vi "NEW数据采集传输系统.vi"() -> ()   [LabVIEW 2016, in "数据传输系统.lvlib"]
uses:
  <vilib>/Utility/miscctls.llb/LVPointTypeDef.ctl
  <vilib>/Utility/error.llb/whitespace.ctl
  <vilib>/picture/picture.llb/imagedata.ctl
  <vilib>/Utility/config.llb/NI_LVConfig.lvlib
  update/update.lvlib
panel:
  in  "串口透传":bool
  in  "共享MN":bool
  out "剖面数据补发":bool
  out "日志信息补发":bool
  out "数据补发":bool
  in  "自动更新":bool
  in  "数据补传":bool caption="确定"
  out "数据库打开失败次数":dbl
  out "与工控通信指示灯":bool
  in  "判断数据反馈":enum16{"非严格判断", "严格判断", "不判断"}(ring)
  in  "暂停上传":bool
  in  "配置表":bool caption="确定"
  in  "updateconfiguration":T1={"主机"="27.154.58.30", "用户"="update", "密码"="std23506", "远程路径"="数据传输系统\\平台数据传输系统.exe", "下载文件名"="平台数据传输系统.exe", "软件版本"=""}
  out "标题显示":string
  in  "更新":bool
  in  "系统编码选择框":string(combo)="地表水质量监测"
  in  "数据发送通道":enum16{"TCP", "VISA"}(ring)
  in  "baud rate":u32=9600 caption="波特率"
  in  "VISA resource name":refnum<visa-resource-name> caption="VISA资源名称"
  in  "实时数据发送时间间隔/min":i32=1
  in  "数据组合发送":bool
  in  "2011发送":bool
  in  "数据发送协议":enum16{"2005-212协议", "2017-212协议"}(ring)=enum."2017-212协议"
  in  "重发时间":T2(ring)
  in  "重发日期":T3(ring)
  in  "开机启动":bool
  in  "每周自动重发":bool=TRUE
  in  "确定":bool
  in  "返回":bool
  in  "PW":string
  in  "MN":string
  in  "PORT":string
  in  "IP":string
  in  "站点设备":string
  in  "站点名称":string
  out "设置超时时间/min":i32=1
  out "状态信息":T4={"1st Error to Convert "=63, "步骤 "=enum."发送数据", "元素"="实时数据", "TCP服务端掉线计数"=0, "TCP掉线时间节点"="2019/05/08 15:24:17"} {"1st Error to Convert" items=["无错误", "参数错误", "内存已满", "超出区域", "文件结束", "文件已打开", "一般文件IO错误", "未找到文件", "文件权限错误", "磁盘已满", "路径副本", "打开过多文件", "未启用", "未找到资源文件", "无法添加资源", "未找到资源", "未找到图像", "图像内存错误", "画笔不存在", "配置错误类型", "配置未找到解析段", "配置解析错误", "配置内存错误", "错误外部代码格式", "错误外部代码偏移量", "外部代码不存在", "空窗口", "销毁窗口错误", "空菜单", "打印已中止", "错误打印记录", "打印驱动程序错误", "打印时窗口错误", "打印时内存错误", "打印对话框错误", "一般打印错误", "无效设备引用句柄", "设备未找到", "设备参数错误", "设备单位错误", "无法打开设备", "设备调用已中止", "一般错误", "用户已取消", "对象ID过低", "对象ID过高", "对象不在堆中", "未知的堆", "错误DefProc ID", "DefProc不在表格中", "范围外信息", "空方法", "未知信息", "不支持管理器调用", "错误地址", "连接过程中", "连接超时", "连接过程中", "不支持网络属性", "网络错误", "正在使用的地址", "系统缺少内存", "连接已中止", "连接已拒绝", "连接未建立", "连接已建立", "连接已关闭", "初始化错误（交互应用程序管理器）", "错误事件发生", "等待无约束事件发生处理程序", "事件发生队列溢出", "错误路径", "未发出信号量", "未识别类型（交互应用程序管理器）"]}
  out "数据接收超时指示灯":bool
  out "空闲时间/s":string
  out "系统时间":string
  out "实时小时数据上传":bool
  out "系统状态改变":bool
  out "软件版本":string
  out "掉线指示":bool
  out "核查数据上传":bool
  out "配置信息":T5
  in  "参数配置":bool
  out "反控数据发送":bool
  out "读取报文显示":string
  out "发送报文显示":string
  out "心跳包":bool
  out "通信状态":bool
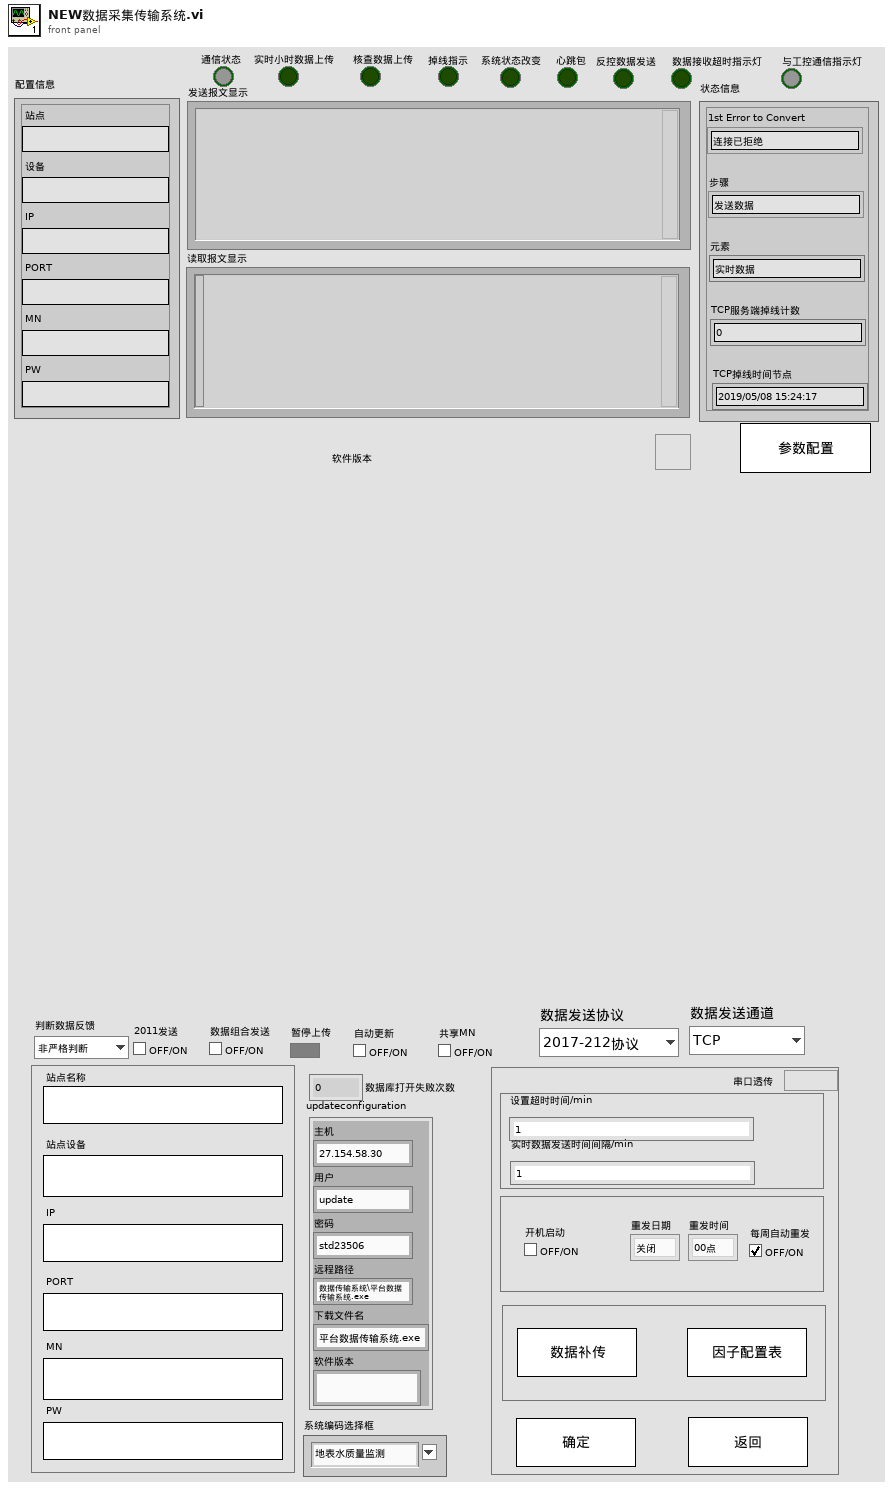
[diagram p1: front panel]
types:
  T1 = cluster{"主机":string, "用户":string, "密码":string, "远程路径":string, "下载文件名":string, "软件版本":string}
  T2 = enum16{"00点", "01点", "02点", "03点", "04点", "05点", "06点", "07点", "08点", "09点", "10点", "11点", "12点", "13点", "14点", "15点", "16点", "17点", "18点", "19点", "20点", "21点", "22点", "23点"}
  T3 = enum16{"关闭", "星期日", "星期一", "星期二", "星期三", "星期四", "星期五", "星期六"}
  T4 = cluster{"1st Error to Convert ":i32, "步骤 ":enum16{"打开连接", "发送数据", "读取数据", "数据处理", "关闭连接"}, "元素":string, "TCP服务端掉线计数":i32, "TCP掉线时间节点":string}
  T5 = cluster{"站点":string, "设备":string, "IP":string, "PORT":string, "MN":string, "PW":string}
  T6 = typedef "imagedata.ctl" = cluster{"image type":i32, "image depth":i32, "image":u8[], "mask":u8[], "colors":u32[], "Rectangle":cluster{"left":i16, "top":i16, "right":i16, "bottom":i16}}
  T7 = typedef "LVPointTypeDef.ctl" = cluster{"Horizontal":i16, "Vertical":i16}
  T8 = cluster{"setini":string, "sysini":string, "hechaini":string, "actualwrite":string, "actualread":string, "datasent":string, "反控命令信息队列":string, "反控与仪器交互":string}
  T9 = cluster{"配置表格[0]":string, "配置表格[1]":string, "配置表格[2]":string, "配置表格[3]":string, "配置表格[4]":string, "配置表格[5]":string, "配置表格[6]":string, "配置表格[7]":string, "配置表格[8]":string, "配置表格[9]":string, "配置表格[10]":string, "配置表格[11]":string, "配置表格[12]":string, "配置表格[13]":string, "配置表格[14]":string, "配置表格[15]":string, "配置表格[16]":string, "配置表格[17]":string, "配置表格[18]":string, "配置表格[19]":string, "配置表格[20]":string, "配置表格[21]":string, "配置表格[22]":string, "配置表格[23]":string, "配置表格[24]":string, "配置表格[25]":string, "配置表格[26]":string, "配置表格[27]":string, "配置表格[28]":string, "配置表格[29]":string, "配置表格[30]":string, "配置表格[31]":string, "配置表格[32]":string, "配置表格[33]":string, "配置表格[34]":string, "配置表格[35]":string, "配置表格[36]":string, "配置表格[37]":string}
  T10 = cluster{"[0]":dbl, "[1]":dbl, "[2]":dbl, "[3]":dbl, "[4]":dbl, "[5]":dbl, "[6]":dbl, "[7]":dbl, "[8]":dbl, "[9]":dbl, "[10]":dbl, "[11]":dbl, "[12]":dbl, "[13]":dbl, "[14]":dbl, "[15]":dbl, "[16]":dbl, "[17]":dbl, "[18]":dbl, "[19]":dbl, "[20]":dbl, "[21]":dbl, "[22]":dbl, "[23]":dbl, "[24]":dbl, "[25]":dbl, "[26]":dbl, "[27]":dbl, "[28]":dbl, "[29]":dbl, "[30]":dbl, "[31]":dbl, "[32]":dbl, "[33]":dbl, "[34]":dbl, "[35]":dbl, "[36]":dbl, "[37]":dbl}
  T11 = cluster{"时间标识":timestamp, "设备":string, "日志信息":string, "流程参数":string}
  T12 = typedef "NI_LVConfig.lvlib/Config Data RefNum.ctl" = refnum<k1>
  T13 = cluster{"CODMn":bool, "CODCr":bool, "DO":bool, "铜":bool, "PH":bool, "氨氮":bool, "比电导率":bool, "水温":bool, "COD":bool, "浊度":bool, "总氮":bool, "总磷":bool, "叶绿素a":bool, "藻密度":bool, "水位":bool, "流速":bool, "瞬时流量":bool, "累积流量":bool, "亚硝氮":bool, "硫化物":bool, "ORP":bool, "铅":bool, "镉":bool, "锌":bool, "镍":bool, "锰":bool, "汞":bool, "气温":bool, "气压":bool, "风速":bool, "风向":bool, "盐度":bool, "磷酸盐":bool, "硝氮":bool, "氟化物":bool, "挥发酚":bool, "氯化物":bool}
  T14 = cluster{"time1":string, "time2":string, "time3":string, "time4":string, "time5":string, "time6":string, "time7":string, "time8":string, "time9":string, "time10":string, "time11":string, "time12":string, "time13":string, "time14":string, "time15":string, "time16":string, "time17":string, "time18":string, "time19":string, "time20":string, "time21":string, "time22":string, "time23":string, "time24":string, "time25":string, "time26":string, "time27":string, "time28":string, "time29":string, "time30":string, "time31":string, "time32":string, "time33":string, "time34":string, "time35":string, "time36":string, "time37":string}
  T15 = cluster{"[0]":string, "[1]":string, "[2]":string, "[3]":string, "[4]":string, "[5]":string, "[6]":string, "[7]":string}
  T16 = cluster{"[0]":string, "[1]":string, "[2]":string, "[3]":string, "[4]":string, "[5]":string, "[6]":string, "[7]":string, "[8]":string, "[9]":string}
  T17 = cluster{"[0]":string, "[1]":string, "[2]":string, "[3]":string, "[4]":string, "[5]":string, "[6]":string}
  T18 = cluster{"[0]":string, "[1]":string, "[2]":string, "[3]":string, "[4]":string, "[5]":string, "[6]":string, "[7]":string, "[8]":string, "[9]":string, "[10]":string, "[11]":string, "[12]":string, "[13]":string, "[14]":string, "[15]":string, "[16]":string, "[17]":string}
  T19 = cluster{"[0]":string, "[1]":string, "[2]":string, "[3]":string, "[4]":string, "[5]":string, "[6]":string, "[7]":string, "[8]":string, "[9]":string, "[10]":string, "[11]":string, "[12]":string, "[13]":string, "[14]":string}
  T20 = cluster{"[0]":string, "[1]":string, "[2]":string, "[3]":string, "[4]":string, "[5]":string, "[6]":string, "[7]":string, "[8]":string, "[9]":string, "[10]":string, "[11]":string, "[12]":string, "[13]":string, "[14]":string, "[15]":string, "[16]":string, "[17]":string, "[18]":string, "[19]":string, "[20]":string, "[21]":string, "[22]":string, "[23]":string, "[24]":string, "[25]":string, "[26]":string, "[27]":string, "[28]":string, "[29]":string, "[30]":string, "[31]":string, "[32]":string, "[33]":string, "[34]":string, "[35]":string, "[36]":string}
  T21 = typedef "whitespace.ctl" = u16
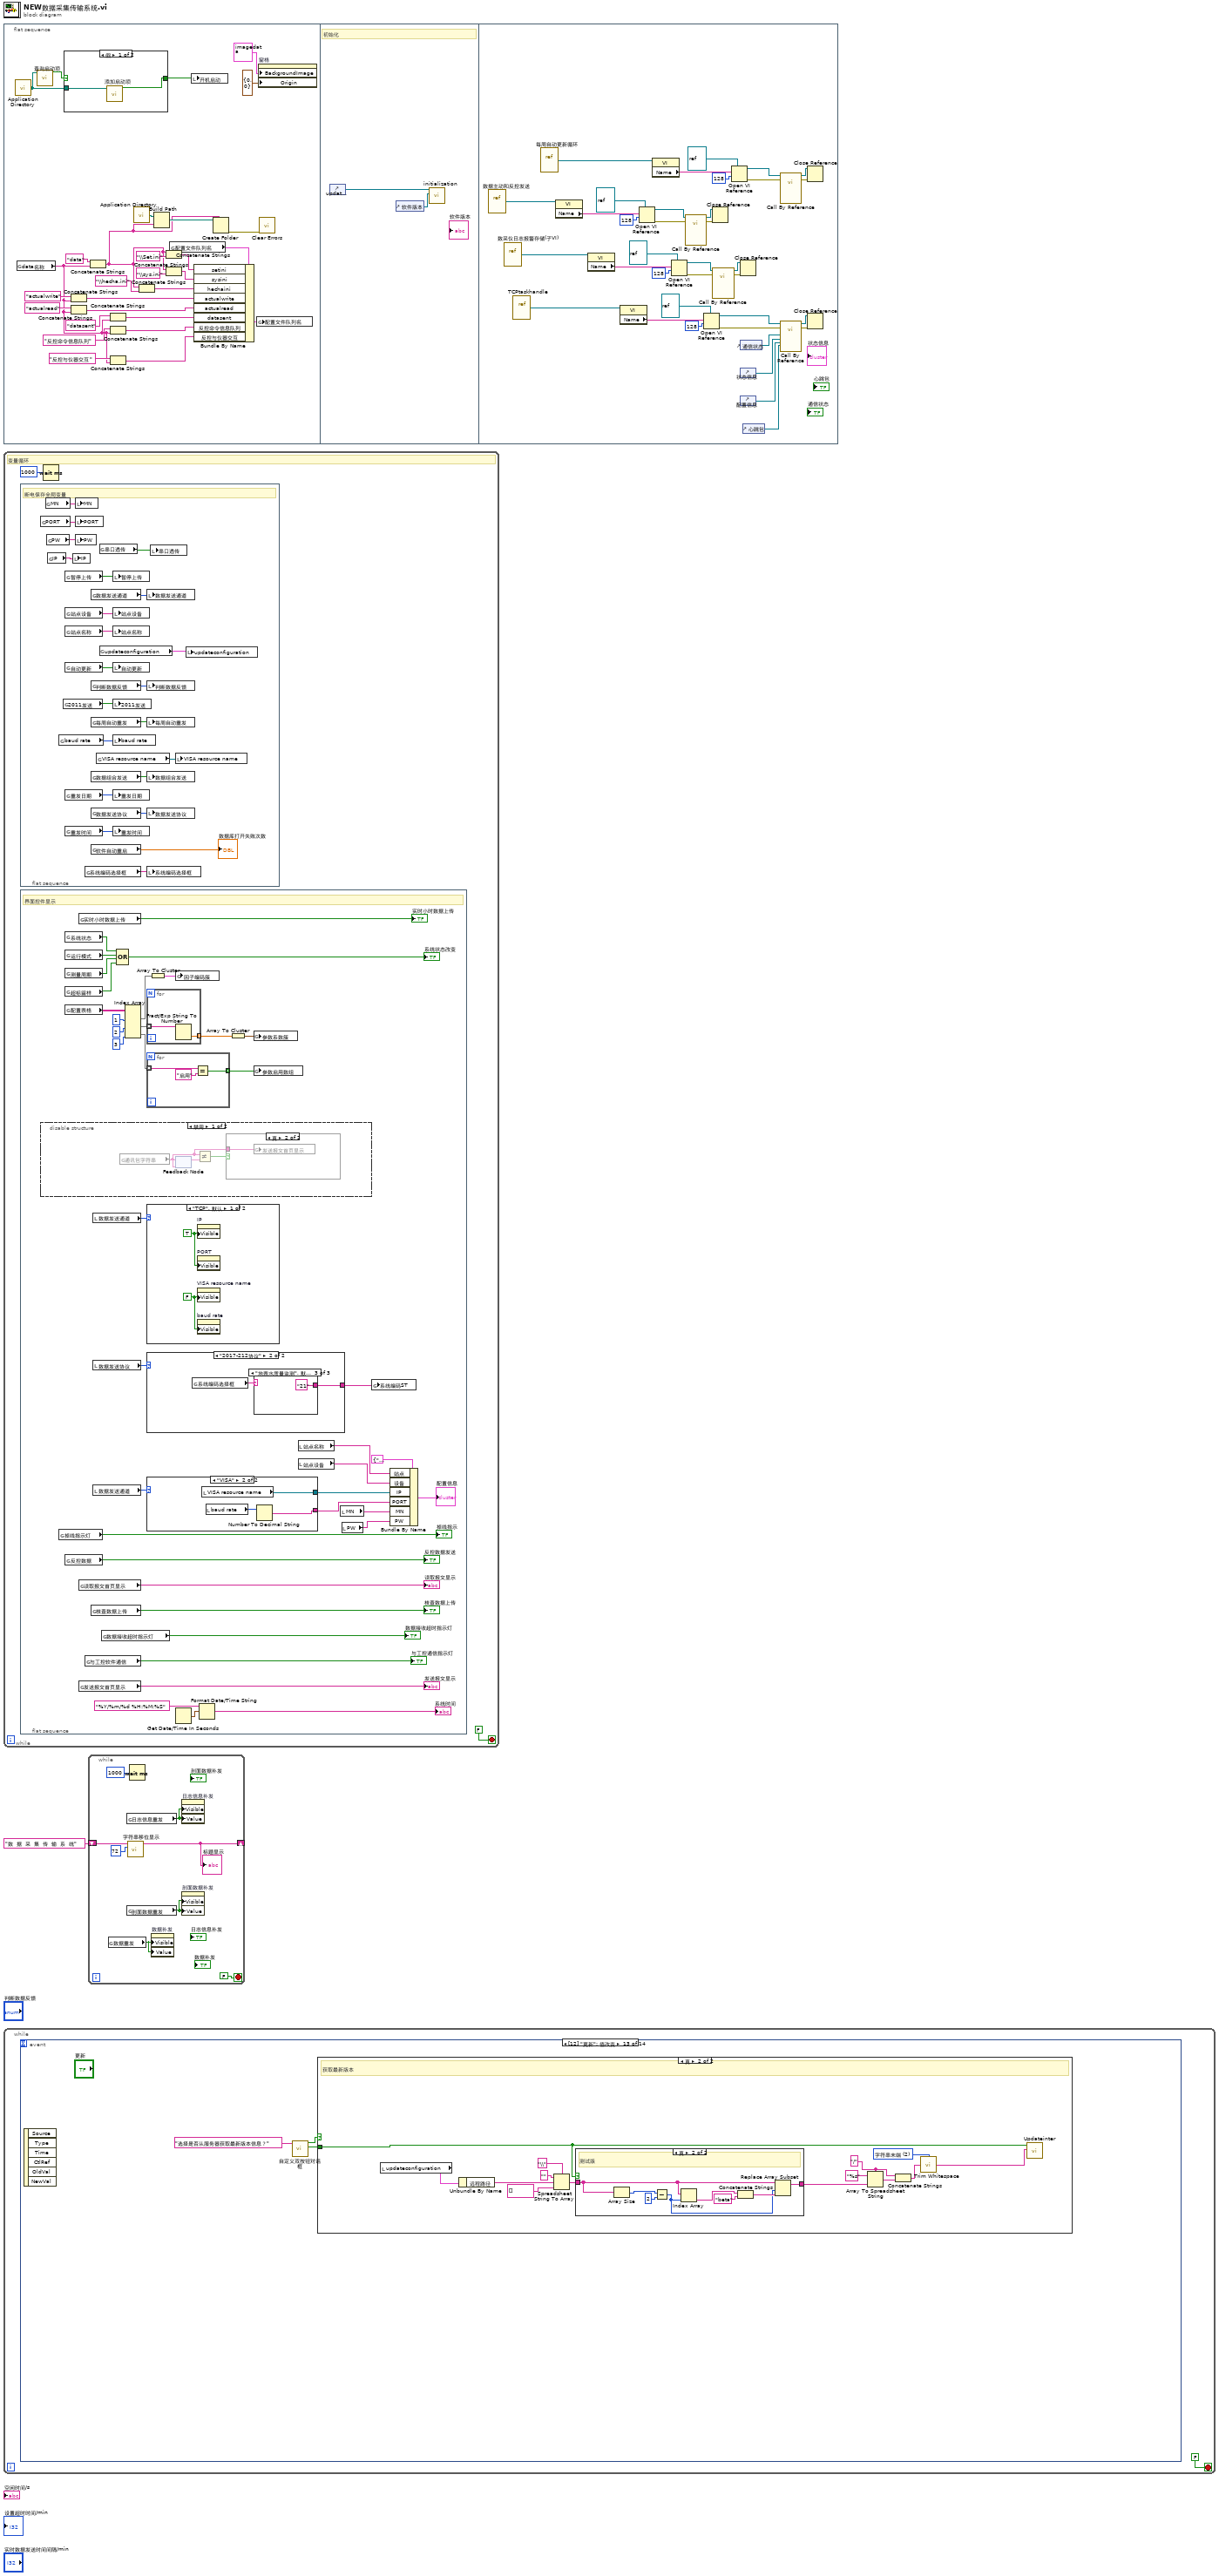
[diagram p0: block diagram]
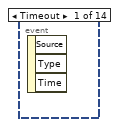
[diagram p2: hidden frame]
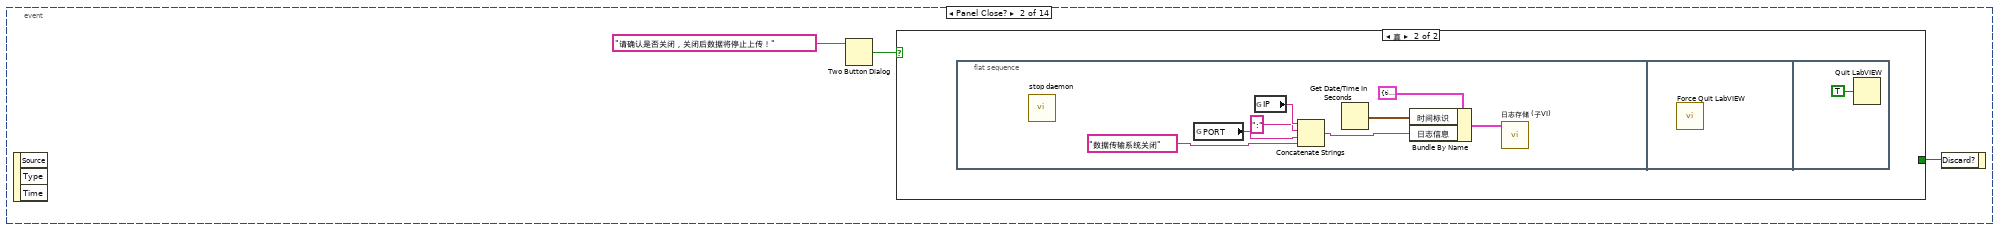
[diagram p3: hidden frame]
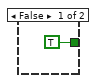
[diagram p4: hidden frame]
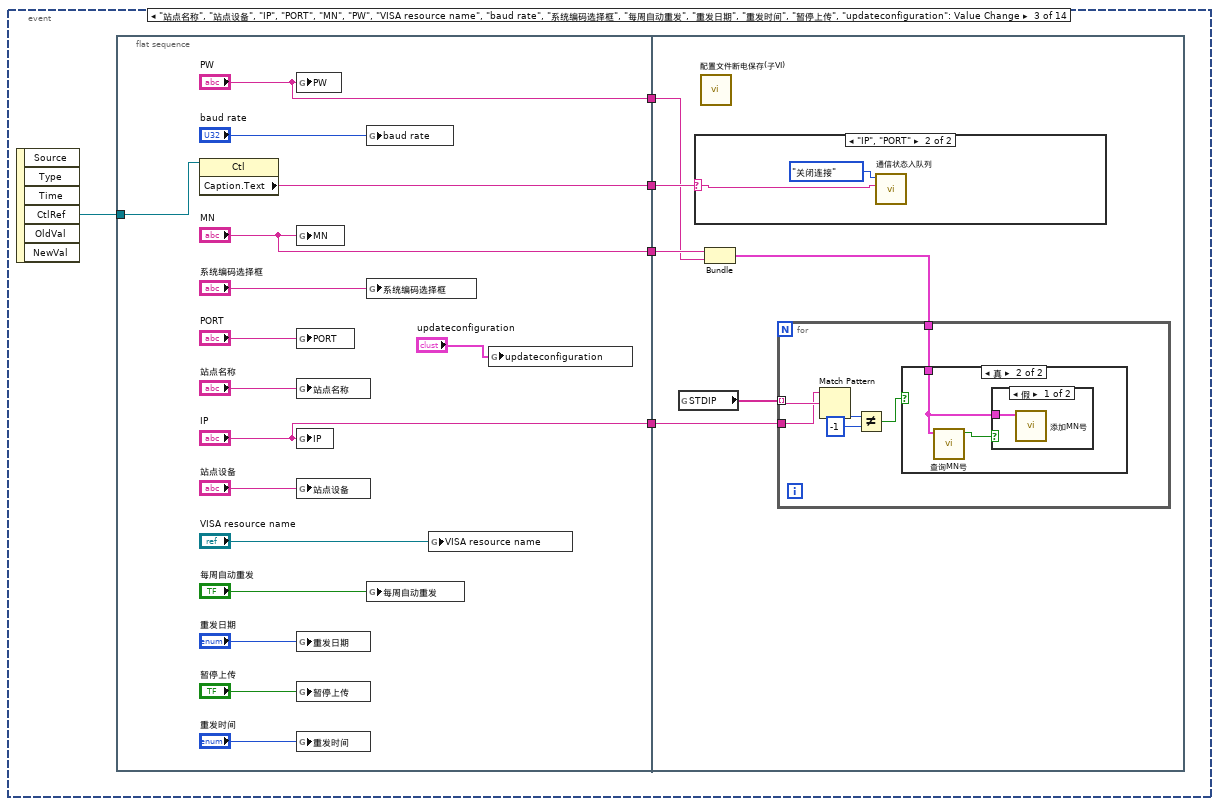
[diagram p5: hidden frame]
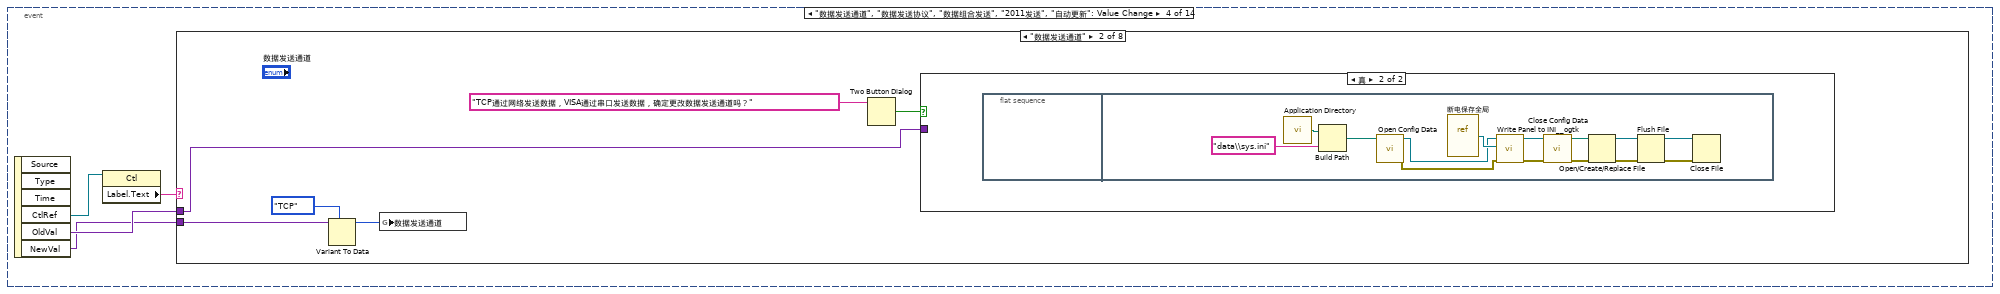
[diagram p9: hidden frame]
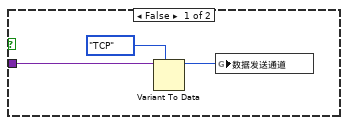
[diagram p11: hidden frame]
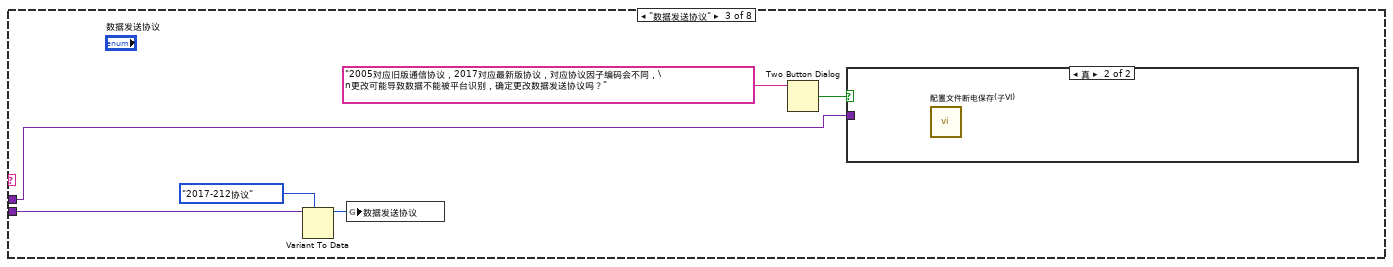
[diagram p12: hidden frame]
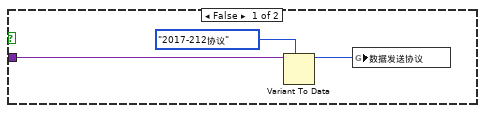
[diagram p13: hidden frame]
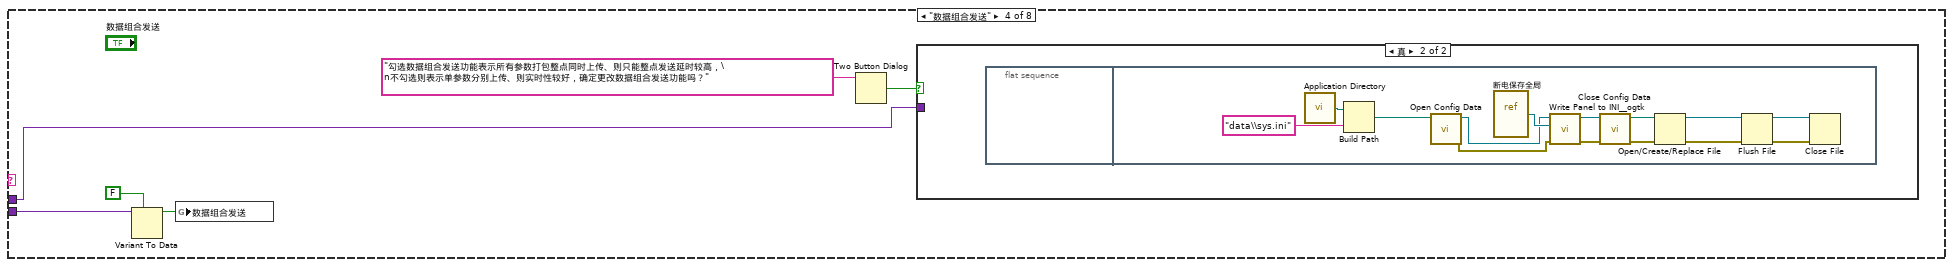
[diagram p14: hidden frame]
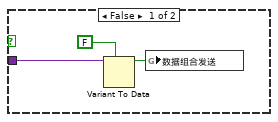
[diagram p15: hidden frame]
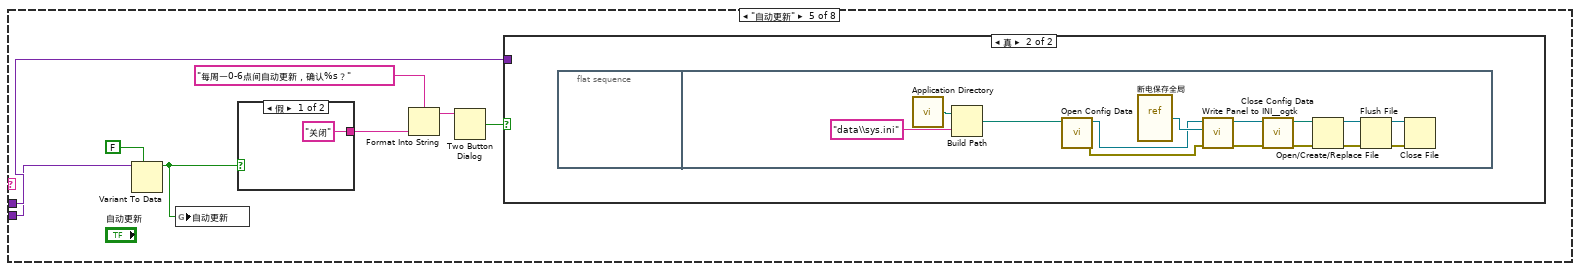
[diagram p16: hidden frame]
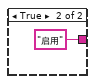
[diagram p17: hidden frame]
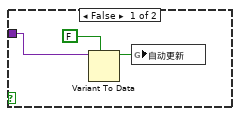
[diagram p18: hidden frame]
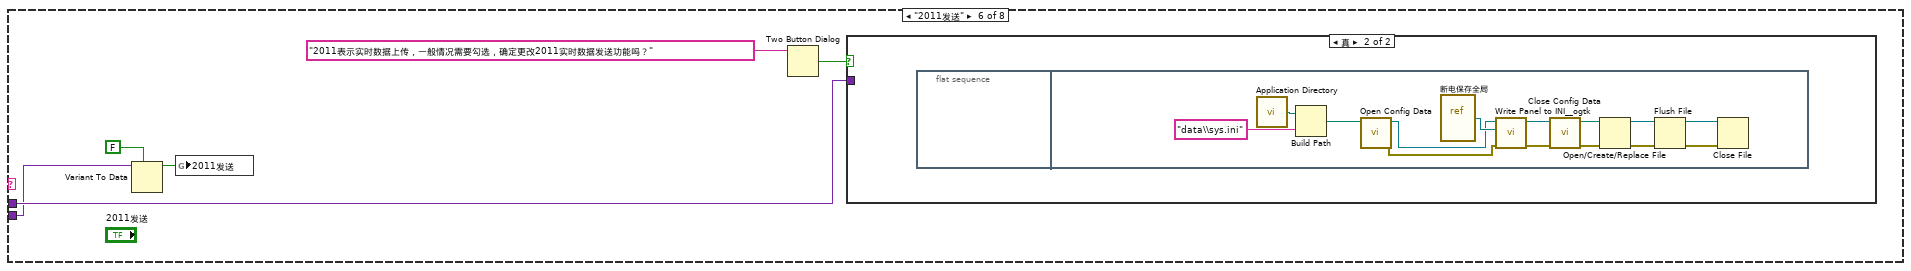
[diagram p19: hidden frame]
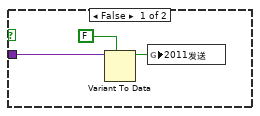
[diagram p20: hidden frame]
diagram:
  n1 = flat-sequence {
    frame #0 {
      n2 = call <vilib>:"Application Directory.vi"() -> ("Application Directory"=w8:path)
      n3 = global read "断电保存全局.vi" "data名称"() -> (w4:string)
      n4 = call "查询启动项.vi"("启动文件路径"=w8) -> ("包含启动项"=w7:bool)  [unwired: 9 in, 1 out]
      n5 = case shown="假" w7 {
        selector: w7 -> [_ w33]
        tunnel: w8 -> [w32 _]
        tunnel: [w31 w33] -> w6
        frame False {
          n6 = call "添加启动项.vi"("启动文件路径"=w32) -> ("添加成功标记"=w31:bool)  [unwired: 9 in, 1 out]
        }
        frame True {
        }
      }
      n7 = Concatenate Strings("actualwrite" ("名称（未命名）"), w4) -> (w18:string)
      n8 = Concatenate Strings("actualread" ("名称（未命名）"), w4) -> (w16:string)
      n9 = Concatenate Strings("data" ("对话框窗口（创建文件夹）"), w4) -> (w23:string)
      n10 = Concatenate Strings("datasent" ("名称（未命名）"), w4) -> (w14:string)
      n11 = Concatenate Strings("反控命令信息队列" ("名称（未命名）"), w4) -> (w10:string)
      n12 = Concatenate Strings("反控与仪器交互" ("名称（未命名）"), w4) -> (w11:string)
      n13 = call <vilib>:"Application Directory.vi"() -> ("Application Directory"=w29:path)
      n14 = Concatenate Strings(w23, "\\hecha.ini" ("名称或相对路径")) -> (w21:string)
      n15 = Build Path(base path=w29, name or relative path=w23) -> (appended path=w28:path)
      n16 = Concatenate Strings(w23, "\\Set.ini" ("名称或相对路径")) -> (w25:string)
      n17 = Concatenate Strings(w23, "\\sys.ini" ("名称或相对路径")) -> (w22:string)
      n18 = global read "全局1.vi" "配置文件队列名"() -> (w2:T8)
      n19 = local write "开机启动"(w6) -> ()
      n20 = Bundle By Name(cluster=w2, "setini"=w25, "sysini"=w22, "hechaini"=w21, "actualwrite"=w18, "actualread"=w16, "datasent"=w14, "反控命令信息队列"=w10, "反控与仪器交互"=w11) -> (w3:T8)
      n21 = Create Folder(prompt (Create Folder)=w23, path (use dialog)=w28) -> (error out=w27:errorcluster)  [unwired: 1 in, 2 out]
      n22 = global write "全局1.vi" "配置文件队列名"(w3) -> ()
      n23 = property on="窗格" class="Pane"("BackgroundImage"=T6 {"image type"=0, "image depth"=24, "image"=array[12288000 elements], "mask"=[], "colors"=[], "Rectangle"={"left"=0, "top"=0, "right"=2560, "bottom"=1600}} ("image data"), "Origin"=T7 {"Horizontal"=0, "Vertical"=0} ("原点")) -> ()  [unwired: 2 in, 2 out]
      n24 = call <vilib>:"Clear Errors.vi"("error in (no error)"=w27) -> ()  [unwired: 5 in, 2 out]
    }
    frame #1 {
      # "初始化"
      n25 = control-ref of="updateconfiguration"() -> (w35:refnum<vi>)
      n26 = control-ref of="软件版本"() -> (w34:refnum<vi>)
      n27 = call "initialization.vi"("软件版本"=w34, "updateconfiguration"=w35) -> ()  [unwired: 9 in]
    }
    frame #2 {
      n28 = vi-ref "数据主动和反控发送.vi"() -> (w63:refnum<vi>)
      n29 = vi-ref "数采仪日志报警存储(子VI).vi"() -> (w64:refnum<vi>)
      n30 = vi-ref "TCPtaskhandle.vi"() -> (w40:refnum<vi>)
      n31 = vi-ref "每周自动更新循环.vi"() -> (w55:refnum<vi>)
      n32 = property class="VI"(reference=w63) -> ("Name"=w62:string)  [unwired: 1 in, 2 out]
      n33 = property class="VI"(reference=w64) -> ("Name"=w71:string)  [unwired: 1 in, 2 out]
      n34 = property class="VI"(reference=w40) -> ("Name"=w47:string)  [unwired: 1 in, 2 out]
      n35 = Open VI Reference(type specifier VI Refnum (for type only)=refnum<vi> refnum, vi path=w62, options=128 ("选项")) -> (vi reference=w60:refnum<vi>, error out=w58:errorcluster)  [unwired: 3 in]
      n36 = property class="VI"(reference=w55) -> ("Name"=w48:string)  [unwired: 1 in, 2 out]
      n37 = Open VI Reference(type specifier VI Refnum (for type only)=refnum<vi> refnum, vi path=w71, options=128 ("选项")) -> (vi reference=w69:refnum<vi>, error out=w67:errorcluster)  [unwired: 3 in]
      n38 = call-by-ref "?"(reference=w60, error in=w58) -> (reference out=w56:refnum<vi>, error out=w57:errorcluster)  [unwired: 12 in]
      n39 = Open VI Reference(type specifier VI Refnum (for type only)=refnum<vi> refnum, vi path=w47, options=128 ("选项")) -> (vi reference=w45:refnum<vi>, error out=w43:errorcluster)  [unwired: 3 in]
      n40 = Close Reference(reference=w56, error in (no error)=w57) -> ()  [unwired: 1 out]
      n41 = call-by-ref "?"(reference=w69, error in=w67) -> (reference out=w65:refnum<vi>, error out=w66:errorcluster)  [unwired: 12 in]
      n42 = Open VI Reference(type specifier VI Refnum (for type only)=refnum<vi> refnum, vi path=w48, options=128 ("选项")) -> (vi reference=w50:refnum<vi>, error out=w52:errorcluster)  [unwired: 3 in]
      n43 = Close Reference(reference=w65, error in (no error)=w66) -> ()  [unwired: 1 out]
      n44 = control-ref of="通信状态"() -> (w39:refnum<vi>)
      n45 = control-ref of="状态信息"() -> (w38:refnum<vi>)
      n46 = control-ref of="配置信息"() -> (w37:refnum<vi>)
      n47 = control-ref of="心跳包"() -> (w36:refnum<vi>)
      n48 = call-by-ref "?"(reference=w50, error in=w52) -> (reference out=w54:refnum<vi>, error out=w53:errorcluster)  [unwired: 12 in]
      n49 = call-by-ref "?"(reference=w45, error in=w43, "心跳包"=w36, "配置信息"=w37, "状态信息"=w38, "通信状态"=w39) -> (reference out=w41:refnum<vi>, error out=w42:errorcluster)  [unwired: 8 in]
      n50 = Close Reference(reference=w54, error in (no error)=w53) -> ()  [unwired: 1 out]
      n51 = Close Reference(reference=w41, error in (no error)=w42) -> ()  [unwired: 1 out]
    }
  }
  n52 = while {
    stop <- FALSE stop-if-true
    # "变量循环"
    n53 = flat-sequence {
      frame #0 {
        # "断电保存全局变量"
        n54 = global read "断电保存全局.vi" "PORT"() -> (w159:string)
        n55 = global read "断电保存全局.vi" "MN"() -> (w158:string)
        n56 = global read "断电保存全局.vi" "PW"() -> (w157:string)
        n57 = global read "断电保存全局.vi" "IP"() -> (w160:string)
        n58 = global read "断电保存全局.vi" "baud rate"() -> (w155:u32)
        n59 = global read "断电保存全局.vi" "2011发送"() -> (w151:bool)
        n60 = global read "断电保存全局.vi" "暂停上传"() -> (w145:bool)
        n61 = global read "断电保存全局.vi" "站点设备"() -> (w161:string)
        n62 = global read "断电保存全局.vi" "站点名称"() -> (w162:string)
        n63 = global read "断电保存全局.vi" "自动更新"() -> (w143:bool)
        n64 = global read "断电保存全局.vi" "重发日期"() -> (w153:T3)
        n65 = global read "断电保存全局.vi" "重发时间"() -> (w146:T2)
        n66 = local write "IP"(w160) -> ()
        n67 = local write "MN"(w158) -> ()
        n68 = local write "PORT"(w159) -> ()
        n69 = local write "PW"(w157) -> ()
        n70 = global read "断电保存全局.vi" "系统编码选择框"() -> (w147:string)
        n71 = global read "断电保存全局.vi" "数据发送通道"() -> (w148:enum16{"TCP", "VISA"})
        n72 = global read "断电保存全局.vi" "判断数据反馈"() -> (w152:enum16{"非严格判断", "严格判断", "不判断"})
        n73 = global read "断电保存全局.vi" "每周自动重发"() -> (w154:bool)
        n74 = global read "断电保存全局.vi" "数据组合发送"() -> (w150:bool)
        n75 = global read "断电保存全局.vi" "数据发送协议"() -> (w149:enum16{"2005-212协议", "2017-212协议"})
        n76 = global read "全局1.vi" "软件自动重启"() -> (→"数据库打开失败次数":dbl)
        n77 = global read "断电保存全局.vi" "VISA resource name"() -> (w156:refnum<visa-resource-name>)
        n78 = global read "断电保存全局.vi" "串口透传"() -> (w141:bool)
        n79 = global read "断电保存全局.vi" "updateconfiguration"() -> (w142:T1)
        n80 = local write "暂停上传"(w145) -> ()
        n81 = local write "站点设备"(w161) -> ()
        n82 = local write "站点名称"(w162) -> ()
        n83 = local write "自动更新"(w143) -> ()
        n84 = local write "2011发送"(w151) -> ()
        n85 = local write "baud rate"(w155) -> ()
        n86 = local write "重发日期"(w153) -> ()
        n87 = local write "重发时间"(w146) -> ()
        n88 = local write "数据发送通道"(w148) -> ()
        n89 = local write "判断数据反馈"(w152) -> ()
        n90 = local write "每周自动重发"(w154) -> ()
        n91 = local write "数据组合发送"(w150) -> ()
        n92 = local write "数据发送协议"(w149) -> ()
        n93 = local write "系统编码选择框"(w147) -> ()
        n94 = local write "串口透传"(w141) -> ()
        n95 = local write "VISA resource name"(w156) -> ()
        n96 = local write "updateconfiguration"(w142) -> ()
      }
    }
    n97 = flat-sequence {
      frame #0 {
        # "界面控件显示"
        n98 = disable-structure shown="禁用" {
          frame Disabled {
            n99 = global read "全局1.vi" "通讯包字符串"() -> (w114:string)
            n100 = feedback #1(w114) -> (w115:string)
            n101 = feedback-in #1(w114) -> ()
            n102 = Not Equal?(x=w114, y=w115) -> (x != y?=w113:bool)
            n103 = case shown="真" w113 {
              tunnel: w114 -> [_ w116]
              frame False {
              }
              frame True {
                n104 = global write "全局1.vi" "发送报文首页显示"(w116) -> ()
              }
            }
          }
          frame Enabled {
          }
        }
        n105 = global read "全局 数据发送重叠.vi" "掉线指示灯"() -> (→"掉线指示":bool)
        n106 = global read "全局1.vi" "系统状态"() -> (w86:bool)
        n107 = global read "全局1.vi" "运行模式"() -> (w87:bool)
        n108 = global read "全局1.vi" "测量周期"() -> (w88:bool)
        n109 = global read "全局1.vi" "超标留样"() -> (w89:bool)
        n110 = global read "断电保存全局.vi" "配置表格"() -> (w84:string[][])
        n111 = global read "全局1.vi" "反控数据"() -> (→"反控数据发送":bool)
        n112 = global read "全局1.vi" "实时小时数据上传"() -> (→"实时小时数据上传":bool)
        n113 = global read "全局1.vi" "读取报文首页显示"() -> (→"读取报文显示":string)
        n114 = global read "全局1.vi" "发送报文首页显示"() -> (→"发送报文显示":string)
        n115 = global read "全局1.vi" "与工控软件通信"() -> (→"与工控通信指示灯":bool)
        n116 = global read "全局1.vi" "核查数据上传"() -> (→"核查数据上传":bool)
        n117 = local read "数据发送通道"() -> (w94:enum16{"TCP", "VISA"})
        n118 = local read "数据发送协议"() -> (w101:enum16{"2005-212协议", "2017-212协议"})
        n119 = local read "数据发送通道"() -> (w112:enum16{"TCP", "VISA"})
        n120 = global read "全局 数据发送重叠.vi" "数据接收超时指示灯"() -> (→"数据接收超时指示灯":bool)
        n121 = Compound Arithmetic op=OR ("复合运算")(w86, w87, w88, w89) -> (→"系统状态改变":bool)
        n122 = Index Array(array=w84, index (col) #1=1 ("禁用的索引 (列)"), index (col) #2=2 ("索引 (列)"), index (col) #3=3 ("索引 (列)")) -> (element #1=w82:string[], element #2=w76:string[], element #3=w78:string[])  [unwired: 3 in]
        n123 = for {
          tunnel: w76 -> [w118] mode=indexing
          tunnel: [w117] -> w75 mode=indexing
          n124 = Fract/Exp String To Number(string=w118) -> (number=w117:dbl)  [unwired: 3 in, 1 out]
        }
        n125 = for {
          tunnel: w78 -> [w121] mode=indexing
          tunnel: [w119] -> w77 mode=indexing
          n126 = Equal?(x=w121, y="启用") -> (x = y?=w119:bool)
        }
        n127 = case shown="\"TCP\", 默认" w94 {
          frame "TCP", Default {
            w122 = TRUE ("可见")
            w123 = FALSE ("可见")
            n128 = property on="IP" class="Str"("Visible"=w122) -> ()  [unwired: 2 in, 2 out]
            n129 = property on="PORT" class="Str"("Visible"=w122) -> ()  [unwired: 2 in, 2 out]
            n130 = property on="VISA resource name" class="VISAName"("Visible"=w123) -> ()  [unwired: 2 in, 2 out]
            n131 = property on="baud rate" class="DigNum (严格)"("Visible"=w123) -> ()  [unwired: 2 in, 2 out]
          }
          frame "VISA" {
            w124 = FALSE ("可见")
            w125 = TRUE ("可见")
            n132 = property on="IP" class="Str"("Visible"=w124) -> ()  [unwired: 2 in, 2 out]
            n133 = property on="PORT" class="Str"("Visible"=w124) -> ()  [unwired: 2 in, 2 out]
            n134 = property on="VISA resource name" class="VISAName"("Visible"=w125) -> ()  [unwired: 2 in, 2 out]
            n135 = property on="baud rate" class="DigNum (严格)"("Visible"=w125) -> ()  [unwired: 2 in, 2 out]
          }
        }
        n136 = case shown="\"2017-212协议\"" w101 {
          tunnel: [w126 w131] -> w100
          frame "2005-212协议", Default {
            n137 = global read "断电保存全局.vi" "系统编码选择框"() -> (w127:string)
            n138 = case shown="\"地表水体污染源\"" w127 {
              tunnel: ["52" ("设备编码MN") "32" ("设备编码MN") "21" ("设备编码MN")] -> w126
              frame "污水排放过程监测" {
              }
              frame "地表水体污染源" {
              }
              frame "地表水质量监测", Default {
              }
            }
          }
          frame "2017-212协议" {
            n139 = global read "断电保存全局.vi" "系统编码选择框"() -> (w132:string)
            n140 = case shown="\"地表水质量监测\", 默认" w132 {
              tunnel: ["52" ("设备编码MN") "32" ("设备编码MN") "21" ("设备编码MN")] -> w131
              frame "污水排放过程监测" {
              }
              frame "地表水体污染源" {
              }
              frame "地表水质量监测", Default {
              }
            }
          }
        }
        n141 = case shown="\"VISA\"" w112 {
          tunnel: [w137 w140] -> w109
          tunnel: [w136 w138] -> w106
          frame "TCP", Default {
            n142 = local read "PORT"() -> (w136:string)
            n143 = local read "IP"() -> (w137:string)
          }
          frame "VISA" {
            n144 = local read "VISA resource name"() -> (w140:refnum<visa-resource-name>)
            n145 = local read "baud rate"() -> (w139:u32)
            n146 = Number To Decimal String(number=w139) -> (decimal integer string=w138:string)  [unwired: 1 in]
          }
        }
        n147 = Array To Cluster(array=w82) -> (cluster=w85:T9)
        n148 = global write "断电保存全局.vi" "因子编码簇"(w85) -> ()
        n149 = Get Date/Time In Seconds() -> (seconds since 1Jan1904=w102:timestamp)
        n150 = Format Date/Time String(time format string (%c)="%Y/%m/%d %H:%M:%S" ("时间格式字符串(%c)"), seconds (now)=w102) -> (date/time string=→"系统时间":string)  [unwired: 1 in]
        n151 = Array To Cluster(array=w75) -> (cluster=w79:T10)
        n152 = global write "断电保存全局.vi" "参数系数簇"(w79) -> ()
        n153 = global write "断电保存全局.vi" "参数启用数组"(w77) -> ()
        n154 = local read "站点名称"() -> (w108:string)
        n155 = local read "站点设备"() -> (w107:string)
        n156 = local read "MN"() -> (w105:string)
        n157 = local read "PW"() -> (w104:string)
        n158 = global write "全局1.vi" "系统编码ST"(w100) -> ()
        n159 = Bundle By Name(cluster=T5 {"站点"="", "设备"="", "IP"="", "PORT"="", "MN"="", "PW"=""} ("配置信息"), "站点"=w108, "设备"=w107, "IP"=w109, "PORT"=w106, "MN"=w105, "PW"=w104) -> (→"配置信息":T5)
      }
    }
    n160 = Wait (ms)(milliseconds to wait=u32 1000 ("等待时间（毫秒）")) -> ()  [unwired: 1 out]
  }
  n161 = while {
    stop <- FALSE stop-if-true
    n162 = event shown="[12] \"更新\": 值改变" {
      selector: _ -> [_ _ _ _ _ _ _ _ _ _ _ _ _ _]
      dyn-events: _ -> [_ _ _ _ _ _ _ _ _ _ _ _ _ _]
      timeout: _ -> [_ _ _ _ _ _ _ _ _ _ _ _ _ _]
      event Timeout {
        n163 = event-data() -> ()  [unwired: 1 in, 3 out]
      }
      event Panel Close? {
        n164 = event-data() -> ()  [unwired: 1 in, 3 out]
        n165 = Two Button Dialog(message="请确认是否关闭，关闭后数据将停止上传！" ("消息")) -> (T button?=w165:bool)  [unwired: 2 in]
        n166 = case shown="真" w165 {
          tunnel: [TRUE _] -> w164
          frame False {
          }
          frame True {
            n167 = flat-sequence {
              frame #0 {
                n168 = call "stop daemon.vi"() -> ()  [unwired: 11 in, 1 out]
                n169 = global read "断电保存全局.vi" "PORT"() -> (w171:string)
                n170 = global read "断电保存全局.vi" "IP"() -> (w173:string)
                n171 = Concatenate Strings(w173, ":", w171, "数据传输系统关闭" ("日志信息")) -> (w169:string)
                n172 = Get Date/Time In Seconds() -> (seconds since 1Jan1904=w175:timestamp)
                n173 = Bundle By Name(cluster=T11 {"时间标识"=timestamp(0 s since 1904-01-01), "设备"="数采仪", "日志信息"="", "流程参数"=""} ("data in"), "时间标识"=w175, "日志信息"=w169) -> (w174:T11)
                n174 = call "日志存储 (子VI).vi"("data in"=w174) -> ()  [unwired: 11 in]
              }
              frame #1 {
                n175 = call "Force Quit LabVIEW.vi"() -> ()  [unwired: 10 in, 2 out]
              }
              frame #2 {
                n176 = Quit LabVIEW(quit? (T)=TRUE ("退出？(T)")) -> ()
              }
            }
          }
        }
        n177 = event-data("Discard?"=w164) -> ()  [unwired: 1 in, 1 out]
      }
      event "站点名称", "站点设备", "IP", "PORT", "MN", "PW", "VISA resource name", "baud rate", "系统编码选择框", "每周自动重发", "重发日期", "重发时间", "暂停上传", "updateconfiguration": Value Change {
        n178 = event-data() -> ("CtlRef"=w181:refnum<vi>)  [unwired: 1 in, 5 out]
        n179 = flat-sequence {
          tunnel: w181 -> [w187]
          tunnel: [w186] -> w180
          tunnel: ["IP"] -> w179
          tunnel: ["MN"] -> w178
          tunnel: ["PW"] -> w177
          tunnel: w180 -> [w203]
          tunnel: w179 -> [w201]
          tunnel: w178 -> [w200]
          tunnel: w177 -> [w199]
          frame #0 {
            n180 = property class="Ctl"(reference=w187) -> ("Caption.Text"=w186:string)  [unwired: 1 in, 2 out]
            n181 = global write "断电保存全局.vi" "PW"("PW") -> ()
            n182 = global write "断电保存全局.vi" "MN"("MN") -> ()
            n183 = global write "断电保存全局.vi" "PORT"("PORT") -> ()
            n184 = global write "断电保存全局.vi" "站点名称"("站点名称") -> ()
            n185 = global write "断电保存全局.vi" "IP"("IP") -> ()
            n186 = global write "断电保存全局.vi" "站点设备"("站点设备") -> ()
            n187 = global write "断电保存全局.vi" "重发日期"("重发日期") -> ()
            n188 = global write "断电保存全局.vi" "暂停上传"("暂停上传") -> ()
            n189 = global write "断电保存全局.vi" "重发时间"("重发时间") -> ()
            n190 = global write "断电保存全局.vi" "baud rate"("baud rate") -> ()
            n191 = global write "断电保存全局.vi" "系统编码选择框"("系统编码选择框") -> ()
            n192 = global write "断电保存全局.vi" "每周自动重发"("每周自动重发") -> ()
            n193 = global write "断电保存全局.vi" "VISA resource name"("VISA resource name") -> ()
            n194 = global write "断电保存全局.vi" "updateconfiguration"("updateconfiguration") -> ()
          }
          frame #1 {
            n195 = global read "断电保存全局.vi" "STDIP"() -> (w202:string[])
            n196 = case shown="\"IP\", \"PORT\"" w203 {
              selector: w203 -> [_ w213]
              frame "假", Default {
              }
              frame "IP", "PORT" {
                n197 = call "通信状态入队列.vi"("发送报文"=w213, "枚举"=enum16{"打开连接", "发送数据", "读取数据", "数据处理", "关闭连接"}."关闭连接") -> ()  [unwired: 9 in, 1 out]
              }
            }
            n198 = call "配置文件断电保存(子VI).vi"() -> ()  [unwired: 12 in]
            n199 = Bundle("MN"=w200, "PW"=w199) -> (w198:cluster{"MN":string, "PW":string})  [unwired: 1 in]
            n200 = for {
              tunnel: w202 -> [w209] mode=indexing
              tunnel: w201 -> [w208]
              tunnel: w198 -> [w204]
              n201 = Match Pattern(string=w208, regular expression=w209) -> (offset past match=w207:i32)  [unwired: 1 in, 3 out]
              n202 = Not Equal?(x=w207, y=-1) -> (x != y?=w205:bool)
              n203 = case shown="真" w205 {
                tunnel: w204 -> [_ w211]
                frame False {
                }
                frame True {
                  n204 = call "查询MN号.vi"("簇"=w211) -> ("包含启动项"=w210:bool)  [unwired: 9 in, 1 out]
                  n205 = case shown="假" w210 {
                    tunnel: w211 -> [w212 _]
                    frame False {
                      n206 = call "添加MN号.vi"("簇"=w212) -> ()  [unwired: 9 in, 2 out]
                    }
                    frame True {
                    }
                  }
                }
              }
            }
          }
        }
      }
      event "数据发送通道", "数据发送协议", "数据组合发送", "2011发送", "自动更新": Value Change {
        n207 = event-data() -> ("CtlRef"=w218:refnum<vi>, "OldVal"=w216:variant, "NewVal"=w215:variant)  [unwired: 1 in, 3 out]
        n208 = property class="Ctl"(reference=w218) -> ("Label.Text"=w217:string)  [unwired: 1 in, 2 out]
        n209 = case shown="\"数据发送通道\"" w217 {
          tunnel: w216 -> [_ w222 w245 w254 w280 w304 w327 w348]
          tunnel: w215 -> [_ w219 w242 w251 w278 w301 w324 w347]
          frame "假", Default {
          }
          frame "数据发送通道" {
            n210 = Variant To Data(type=enum16{"TCP", "VISA"}."TCP" ("数据发送通道"), Variant=w219) -> (data=w220:enum16{"TCP", "VISA"})  [unwired: 1 in, 1 out]
            n211 = global write "断电保存全局.vi" "数据发送通道"(w220) -> ()
            n212 = Two Button Dialog(message="TCP通过网络发送数据，VISA通过串口发送数据，确定更改数据发送通道吗？" ("消息")) -> (T button?=w223:bool)  [unwired: 2 in]
            n213 = case shown="真" w223 {
              tunnel: w222 -> [w226 _]
              frame False {
                n214 = Variant To Data(type=enum16{"TCP", "VISA"}."TCP" ("数据发送通道"), Variant=w226) -> (data=w225:enum16{"TCP", "VISA"})  [unwired: 1 in, 1 out]
                n215 = global write "断电保存全局.vi" "数据发送通道"(w225) -> ()
              }
              frame True {
                n216 = flat-sequence {
                  frame #0 {
                  }
                  frame #1 {
                    n217 = call <vilib>:"Application Directory.vi"() -> ("Application Directory"=w228:path)
                    n218 = Build Path(base path=w228, name or relative path="data\\sys.ini" ("名称或相对路径")) -> (appended path=w230:path)
                    n219 = call <vilib>:"Open Config Data.vi"("configuration file path"=w230) -> ("error out"=w234:errorcluster, "refnum"=w231:T12)  [unwired: 8 in, 1 out]
                    n220 = vi-ref "断电保存全局.vi"() -> (w232:refnum<vi>)
                    n221 = call <userlib>:"Write Panel to INI__ogtk.vi"("error in (no error)"=w234, "VI ref"=w232, "refnum"=w231) -> ("error out"=w235:errorcluster, "refnum out"=w233:T12)  [unwired: 7 in]
                    n222 = call <vilib>:"Close Config Data.vi"("error in (no error)"=w235, "refnum"=w233) -> ("error out"=w240:errorcluster, "file path"=w241:path)  [unwired: 8 in]
                    n223 = Open/Create/Replace File(file path (use dialog)=w241, error in=w240) -> (refnum out=w237:refnum<file>, error out=w236:errorcluster)  [unwired: 4 in, 1 out]
                    n224 = Flush File(refnum=w237, error in=w236) -> (refnum out=w238:refnum<file>, error out=w239:errorcluster)
                    n225 = Close File(refnum=w238, error in=w239) -> ()  [unwired: 2 out]
                  }
                }
              }
            }
          }
          frame "数据发送协议" {
            n226 = Variant To Data(type=enum16{"2005-212协议", "2017-212协议"}."2017-212协议" ("数据"), Variant=w242) -> (data=w243:enum16{"2005-212协议", "2017-212协议"})  [unwired: 1 in, 1 out]
            n227 = global write "断电保存全局.vi" "数据发送协议"(w243) -> ()
            n228 = Two Button Dialog(message="2005对应旧版通信协议，2017对应最新版协议，对应协议因子编码会不同，\n更改可能导致数据不能被平台识别，确定更改数据发送协议吗？" ("消息")) -> (T button?=w246:bool)  [unwired: 2 in]
            n229 = case shown="真" w246 {
              tunnel: w245 -> [w250 _]
              frame False {
                n230 = Variant To Data(type=enum16{"2005-212协议", "2017-212协议"}."2017-212协议" ("数据"), Variant=w250) -> (data=w248:enum16{"2005-212协议", "2017-212协议"})  [unwired: 1 in, 1 out]
                n231 = global write "断电保存全局.vi" "数据发送协议"(w248) -> ()
              }
              frame True {
                n232 = call "配置文件断电保存(子VI).vi"() -> ()  [unwired: 12 in]
              }
            }
          }
          frame "数据组合发送" {
            n233 = Variant To Data(type=FALSE, Variant=w251) -> (data=w252:bool)  [unwired: 1 in, 1 out]
            n234 = global write "断电保存全局.vi" "数据组合发送"(w252) -> ()
            n235 = Two Button Dialog(message="勾选数据组合发送功能表示所有参数打包整点同时上传、则只能整点发送延时较高，\n不勾选则表示单参数分别上传、则实时性较好，确定更改数据组合发送功能吗？" ("消息")) -> (T button?=w255:bool)  [unwired: 2 in]
            n236 = case shown="真" w255 {
              tunnel: w254 -> [w258 _]
              frame False {
                n237 = Variant To Data(type=FALSE, Variant=w258) -> (data=w257:bool)  [unwired: 1 in, 1 out]
                n238 = global write "断电保存全局.vi" "数据组合发送"(w257) -> ()
              }
              frame True {
                n239 = flat-sequence {
                  frame #0 {
                  }
                  frame #1 {
                    n240 = call <vilib>:"Application Directory.vi"() -> ("Application Directory"=w260:path)
                    n241 = Build Path(base path=w260, name or relative path="data\\sys.ini" ("名称或相对路径")) -> (appended path=w262:path)
                    n242 = call <vilib>:"Open Config Data.vi"("configuration file path"=w262) -> ("error out"=w266:errorcluster, "refnum"=w263:T12)  [unwired: 8 in, 1 out]
                    n243 = vi-ref "断电保存全局.vi"() -> (w264:refnum<vi>)
                    n244 = call <userlib>:"Write Panel to INI__ogtk.vi"("error in (no error)"=w266, "VI ref"=w264, "refnum"=w263) -> ("error out"=w267:errorcluster, "refnum out"=w265:T12)  [unwired: 7 in]
                    n245 = call <vilib>:"Close Config Data.vi"("error in (no error)"=w267, "refnum"=w265) -> ("error out"=w272:errorcluster, "file path"=w273:path)  [unwired: 8 in]
                    n246 = Open/Create/Replace File(file path (use dialog)=w273, error in=w272) -> (refnum out=w269:refnum<file>, error out=w268:errorcluster)  [unwired: 4 in, 1 out]
                    n247 = Flush File(refnum=w269, error in=w268) -> (refnum out=w270:refnum<file>, error out=w271:errorcluster)
                    n248 = Close File(refnum=w270, error in=w271) -> ()  [unwired: 2 out]
                  }
                }
              }
            }
          }
          frame "自动更新" {
            n249 = Variant To Data(type=FALSE, Variant=w278) -> (data=w276:bool)  [unwired: 1 in, 1 out]
            n250 = global write "断电保存全局.vi" "自动更新"(w276) -> ()
            n251 = case shown="假" w276 {
              tunnel: ["关闭" "启用"] -> w275
              frame False {
              }
              frame True {
              }
            }
            n252 = Format Into String(format string="每周一0-6点间自动更新，确认%s？" ("消息"), w275) -> (resulting string=w274:string)  [unwired: 2 in, 1 out]
            n253 = Two Button Dialog(message=w274) -> (T button?=w281:bool)  [unwired: 2 in]
            n254 = case shown="真" w281 {
              tunnel: w280 -> [w285 _]
              frame False {
                n255 = Variant To Data(type=FALSE, Variant=w285) -> (data=w284:bool)  [unwired: 1 in, 1 out]
                n256 = global write "断电保存全局.vi" "自动更新"(w284) -> ()
              }
              frame True {
                n257 = flat-sequence {
                  frame #0 {
                  }
                  frame #1 {
                    n258 = call <vilib>:"Application Directory.vi"() -> ("Application Directory"=w287:path)
                    n259 = Build Path(base path=w287, name or relative path="data\\sys.ini" ("名称或相对路径")) -> (appended path=w289:path)
                    n260 = call <vilib>:"Open Config Data.vi"("configuration file path"=w289) -> ("error out"=w293:errorcluster, "refnum"=w290:T12)  [unwired: 8 in, 1 out]
                    n261 = vi-ref "断电保存全局.vi"() -> (w291:refnum<vi>)
                    n262 = call <userlib>:"Write Panel to INI__ogtk.vi"("error in (no error)"=w293, "VI ref"=w291, "refnum"=w290) -> ("error out"=w294:errorcluster, "refnum out"=w292:T12)  [unwired: 7 in]
                    n263 = call <vilib>:"Close Config Data.vi"("error in (no error)"=w294, "refnum"=w292) -> ("error out"=w299:errorcluster, "file path"=w300:path)  [unwired: 8 in]
                    n264 = Open/Create/Replace File(file path (use dialog)=w300, error in=w299) -> (refnum out=w296:refnum<file>, error out=w295:errorcluster)  [unwired: 4 in, 1 out]
                    n265 = Flush File(refnum=w296, error in=w295) -> (refnum out=w297:refnum<file>, error out=w298:errorcluster)
                    n266 = Close File(refnum=w297, error in=w298) -> ()  [unwired: 2 out]
                  }
                }
              }
            }
          }
          frame "2011发送" {
            n267 = Variant To Data(type=FALSE, Variant=w301) -> (data=w302:bool)  [unwired: 1 in, 1 out]
            n268 = global write "断电保存全局.vi" "2011发送"(w302) -> ()
            n269 = Two Button Dialog(message="2011表示实时数据上传，一般情况需要勾选，确定更改2011实时数据发送功能吗？" ("消息")) -> (T button?=w305:bool)  [unwired: 2 in]
            n270 = case shown="真" w305 {
              tunnel: w304 -> [w308 _]
              frame False {
                n271 = Variant To Data(type=FALSE, Variant=w308) -> (data=w307:bool)  [unwired: 1 in, 1 out]
                n272 = global write "断电保存全局.vi" "2011发送"(w307) -> ()
              }
              frame True {
                n273 = flat-sequence {
                  frame #0 {
                  }
                  frame #1 {
                    n274 = call <vilib>:"Application Directory.vi"() -> ("Application Directory"=w310:path)
                    n275 = Build Path(base path=w310, name or relative path="data\\sys.ini" ("名称或相对路径")) -> (appended path=w312:path)
                    n276 = call <vilib>:"Open Config Data.vi"("configuration file path"=w312) -> ("error out"=w316:errorcluster, "refnum"=w313:T12)  [unwired: 8 in, 1 out]
                    n277 = vi-ref "断电保存全局.vi"() -> (w314:refnum<vi>)
                    n278 = call <userlib>:"Write Panel to INI__ogtk.vi"("error in (no error)"=w316, "VI ref"=w314, "refnum"=w313) -> ("error out"=w317:errorcluster, "refnum out"=w315:T12)  [unwired: 7 in]
                    n279 = call <vilib>:"Close Config Data.vi"("error in (no error)"=w317, "refnum"=w315) -> ("error out"=w322:errorcluster, "file path"=w323:path)  [unwired: 8 in]
                    n280 = Open/Create/Replace File(file path (use dialog)=w323, error in=w322) -> (refnum out=w319:refnum<file>, error out=w318:errorcluster)  [unwired: 4 in, 1 out]
                    n281 = Flush File(refnum=w319, error in=w318) -> (refnum out=w320:refnum<file>, error out=w321:errorcluster)
                    n282 = Close File(refnum=w320, error in=w321) -> ()  [unwired: 2 out]
                  }
                }
              }
            }
          }
          frame "日志、参数发送" {
            n283 = Variant To Data(type=FALSE, Variant=w324) -> (data=w325:bool)  [unwired: 1 in, 1 out]
            n284 = global write "断电保存全局.vi" "日志、参数发送"(w325) -> ()
            n285 = Two Button Dialog(message="选择是否需要仪器日志、状态和告警信息上传，一般情况需要勾选，确定更改日志、参数发送功能吗？" ("消息")) -> (T button?=w328:bool)  [unwired: 2 in]
            n286 = case shown="假" w328 {
              tunnel: w327 -> [w331 _]
              frame False {
                n287 = Variant To Data(type=FALSE, Variant=w331) -> (data=w330:bool)  [unwired: 1 in, 1 out]
                n288 = global write "断电保存全局.vi" "日志、参数发送"(w330) -> ()
              }
              frame True {
                n289 = flat-sequence {
                  frame #0 {
                  }
                  frame #1 {
                    n290 = call <vilib>:"Application Directory.vi"() -> ("Application Directory"=w333:path)
                    n291 = Build Path(base path=w333, name or relative path="data\\sys.ini" ("名称或相对路径")) -> (appended path=w335:path)
                    n292 = call <vilib>:"Open Config Data.vi"("configuration file path"=w335) -> ("error out"=w339:errorcluster, "refnum"=w336:T12)  [unwired: 8 in, 1 out]
                    n293 = vi-ref "断电保存全局.vi"() -> (w337:refnum<vi>)
                    n294 = call <userlib>:"Write Panel to INI__ogtk.vi"("error in (no error)"=w339, "VI ref"=w337, "refnum"=w336) -> ("error out"=w340:errorcluster, "refnum out"=w338:T12)  [unwired: 7 in]
                    n295 = call <vilib>:"Close Config Data.vi"("error in (no error)"=w340, "refnum"=w338) -> ("error out"=w345:errorcluster, "file path"=w346:path)  [unwired: 8 in]
                    n296 = Open/Create/Replace File(file path (use dialog)=w346, error in=w345) -> (refnum out=w342:refnum<file>, error out=w341:errorcluster)  [unwired: 4 in, 1 out]
                    n297 = Flush File(refnum=w342, error in=w341) -> (refnum out=w343:refnum<file>, error out=w344:errorcluster)
                    n298 = Close File(refnum=w343, error in=w344) -> ()  [unwired: 2 out]
                  }
                }
              }
            }
          }
          frame "判断数据反馈" {
            n299 = Two Button Dialog(message="判断数据反馈是针对平台能有反馈的情况，\n1.严格判断反馈-收不到反馈一直重发\n2.非严格判断-重发5次后跳过该数据\n3.不判断反馈针对平台没有反馈的情况\n确定更改判断数据反馈功能吗？" ("消息")) -> (T button?=w349:bool)  [unwired: 2 in]
            n300 = case shown="假" w349 {
              tunnel: w348 -> [_ _]
              tunnel: w347 -> [w352 w354]
              frame False {
                n301 = Variant To Data(type=enum16{"非严格判断", "严格判断", "不判断"}."非严格判断" ("判断数据反馈"), Variant=w352) -> (data=w351:enum16{"非严格判断", "严格判断", "不判断"})  [unwired: 1 in, 1 out]
                n302 = local write "判断数据反馈"(w351) -> ()
              }
              frame True {
                n303 = flat-sequence {
                  tunnel: w354 -> [w355]
                  frame #0 {
                    n304 = Variant To Data(type=enum16{"非严格判断", "严格判断", "不判断"}."非严格判断" ("判断数据反馈"), Variant=w355) -> (data=w357:enum16{"非严格判断", "严格判断", "不判断"})  [unwired: 1 in, 1 out]
                    n305 = global write "断电保存全局.vi" "判断数据反馈"(w357) -> ()
                  }
                  frame #1 {
                    n306 = call <vilib>:"Application Directory.vi"() -> ("Application Directory"=w358:path)
                    n307 = Build Path(base path=w358, name or relative path="data\\sys.ini" ("名称或相对路径")) -> (appended path=w360:path)
                    n308 = call <vilib>:"Open Config Data.vi"("configuration file path"=w360) -> ("error out"=w364:errorcluster, "refnum"=w361:T12)  [unwired: 8 in, 1 out]
                    n309 = vi-ref "断电保存全局.vi"() -> (w362:refnum<vi>)
                    n310 = call <userlib>:"Write Panel to INI__ogtk.vi"("error in (no error)"=w364, "VI ref"=w362, "refnum"=w361) -> ("error out"=w365:errorcluster, "refnum out"=w363:T12)  [unwired: 7 in]
                    n311 = call <vilib>:"Close Config Data.vi"("error in (no error)"=w365, "refnum"=w363) -> ("error out"=w370:errorcluster, "file path"=w371:path)  [unwired: 8 in]
                    n312 = Open/Create/Replace File(file path (use dialog)=w371, error in=w370) -> (refnum out=w367:refnum<file>, error out=w366:errorcluster)  [unwired: 4 in, 1 out]
                    n313 = Flush File(refnum=w367, error in=w366) -> (refnum out=w368:refnum<file>, error out=w369:errorcluster)
                    n314 = Close File(refnum=w368, error in=w369) -> ()  [unwired: 2 out]
                  }
                }
              }
            }
          }
        }
      }
      event "确定": Value Change {
        n315 = event-data() -> ()  [unwired: 1 in, 6 out]
        n316 = call "通信状态入队列.vi"("枚举"=enum16{"打开连接", "发送数据", "读取数据", "数据处理", "关闭连接"}."关闭连接") -> ()  [unwired: 10 in, 1 out]
      }
      event "配置表": Value Change {
        n317 = event-data() -> ()  [unwired: 1 in, 6 out]
        n318 = call "参数配置表.vi"() -> ()  [unwired: 12 in]
      }
      event "串口透传": Value Change {
        n319 = event-data() -> ()  [unwired: 1 in, 6 out]
        n320 = flat-sequence {
          frame #0 {
            n321 = global write "断电保存全局.vi" "串口透传"("串口透传") -> ()
          }
          frame #1 {
            n322 = call "配置文件断电保存(子VI).vi"() -> ()  [unwired: 12 in]
          }
        }
        n323 = call "串口配置.vi"() -> ()  [unwired: 12 in]
      }
      event "参数配置": Value Change {
        n324 = event-data() -> ()  [unwired: 1 in, 6 out]
        n325 = property on="窗格" class="Pane"("Origin"=T7 {"Horizontal"=0, "Vertical"=1000} ("原点")) -> ()  [unwired: 2 in, 2 out]
        n326 = call <vilib>:"Application Directory.vi"() -> ("Application Directory"=w380:path)
        n327 = call "查询启动项.vi"("启动文件路径"=w380) -> ("error out"=w375:errorcluster, "包含启动项"=w379:bool)  [unwired: 9 in]
        n328 = local write "开机启动"(w379) -> ()
        n329 = local read "MN"() -> (w378:string)
        n330 = local read "PW"() -> (w377:string)
        n331 = Bundle("MN"=w378, "PW"=w377) -> (w376:cluster{"MN":string, "PW":string})  [unwired: 1 in]
        n332 = call "查询MN号.vi"("error in (no error)"=w375, "簇"=w376) -> ("包含启动项"=w374:bool)  [unwired: 8 in, 1 out]
        n333 = local write "共享MN"(w374) -> ()
      }
      event "返回": Value Change {
        n334 = event-data() -> ()  [unwired: 1 in, 6 out]
        n335 = property on="窗格" class="Pane"("Origin"=T7 {"Horizontal"=0, "Vertical"=0} ("原点")) -> ()  [unwired: 2 in, 2 out]
      }
      event "数据补传": Value Change {
        n336 = event-data() -> ()  [unwired: 1 in, 6 out]
        n337 = global read "全局1.vi" "数据发送起始时间"() -> (w385:timestamp)
        n338 = call "数据补传对话框.vi"("起始时间"=w385) -> ("参数数值out"=w384:T13, "结束时间输出"=w386:timestamp, "起始时间输出"=w387:timestamp, "输出"=w388:bool, "只补小时数据输出"=w383:bool)  [unwired: 6 in]
        n339 = case shown="真" w388 {
          tunnel: w387 -> [_ w397]
          tunnel: w386 -> [_ w398]
          tunnel: w384 -> [_ w394]
          tunnel: w383 -> [_ w396]
          frame False {
          }
          frame True {
            w395 = TRUE ("数据重发")
            n340 = global read "全局 水样时间.vi" "水样数据索引"() -> (w393:T14)
            n341 = global write "全局1.vi" "数据发送起始时间"(w397) -> ()
            n342 = global write "断电保存全局.vi" "数据重发结束时间"(w398) -> ()
            n343 = Cluster To Array(cluster=w394) -> (array=w392:bool[])
            n344 = global write "断电保存全局.vi" "数据重发"(w395) -> ()
            n345 = Cluster To Array(cluster=w393) -> (array=w391:string[])
            n346 = Format Date/Time String(time format string (%c)="%Y/%m/%d %H:%M:%S" ("时间格式字符串(%c)"), seconds (now)=w397) -> (date/time string=w390:string)  [unwired: 1 in]
            n347 = for {
              tunnel: w392 -> [w404] mode=indexing
              tunnel: w391 -> [w402] mode=indexing
              tunnel: w390 -> [w403]
              tunnel: [w401] -> w389 mode=indexing
              n348 = Select(t=w403, s=w404, f=w402) -> (s? t:f=w401:string)
            }
            n349 = case shown="假" w396 {
              tunnel: w390 -> [w412 _]
              tunnel: w395 -> [w405 _]
              frame False {
                n350 = global read "断电保存全局.vi" "数据组合发送"() -> (w413:bool)
                n351 = global write "全局 水样时间.vi" "剖面数据时间"(w412) -> ()
                n352 = global write "断电保存全局.vi" "数据重发时间戳"(w412) -> ()
                n353 = Initialize Array(w412, 8 ("维数大小")) -> (w408:string[])
                n354 = Initialize Array(w412, 15 ("维数大小")) -> (w409:string[])
                n355 = global write "全局 水样时间.vi" "剖面多参数数据时间"(w412) -> ()
                n356 = case shown="假" w413 {
                  tunnel: w412 -> [w414 _]
                  frame False {
                    n357 = global write "全局 时间2.vi" "标样核查索引起始时间"(w414) -> ()
                    n358 = global write "全局 时间2.vi" "加标回收索引起始时间"(w414) -> ()
                    n359 = global write "全局 时间2.vi" "跨度核查索引起始时间"(w414) -> ()
                    n360 = global write "全局 时间2.vi" "3092日志索引起始时间"(w414) -> ()
                    n361 = global write "全局 时间2.vi" "零点核查索引起始时间"(w414) -> ()
                    n362 = Initialize Array(w414, 10 ("维数大小")) -> (w426:string[])
                    n363 = Initialize Array(w414, 7 ("维数大小")) -> (w418:string[])
                    n364 = Initialize Array(w414, 8 ("维数大小")) -> (w417:string[])
                    n365 = Initialize Array(w414, 18 ("维数大小")) -> (w421:string[])
                    n366 = Array To Cluster(array=w417) -> (cluster=w416:T15)
                    n367 = Array To Cluster(array=w426) -> (cluster=w425:T16)
                    n368 = Array To Cluster(array=w418) -> (cluster=w419:T17)
                    n369 = global write "全局 时间2.vi" "跨度核查索引"(w425) -> ()
                    n370 = global write "全局 时间2.vi" "零点核查索引"(w425) -> ()
                    n371 = global write "全局 时间2.vi" "平行样索引"(w419) -> ()
                    n372 = global write "全局 时间2.vi" "加标回收索引"(w419) -> ()
                    n373 = global write "全局 时间2.vi" "仪器日志索引"(w416) -> ()
                    n374 = Array To Cluster(array=w421) -> (cluster=w422:T18)
                    n375 = global write "全局 时间2.vi" "标样核查索引"(w422) -> ()
                    n376 = global write "全局 时间2.vi" "集成干预索引"(w422) -> ()
                  }
                  frame True {
                  }
                }
                n377 = Array To Cluster(array=w408) -> (cluster=w407:T15)
                n378 = global write "全局 时间2.vi" "仪器日志索引"(w407) -> ()
                n379 = Array To Cluster(array=w409) -> (cluster=w410:T19)
                n380 = global write "断电保存全局.vi" "日志信息重发"(w405) -> ()
                n381 = global write "断电保存全局.vi" "剖面数据重发"(w405) -> ()
                n382 = global write "全局 时间2.vi" "仪器参数索引"(w410) -> ()
              }
              frame True {
                n383 = global write "断电保存全局.vi" "2011发送"(FALSE ("2011发送")) -> ()
              }
            }
            n384 = Array To Cluster(array=w389) -> (cluster=w399:T20)
            n385 = global write "全局 水样时间.vi" "水样数据索引"(w399) -> ()
          }
        }
      }
      event "开机启动": Value Change {
        n386 = event-data() -> ("CtlRef"=w429:refnum<vi>, "OldVal"=w428:bool, "NewVal"=w430:bool)  [unwired: 1 in, 3 out]
        n387 = case shown="假" w430 {
          tunnel: w429 -> [w432 w445]
          tunnel: w428 -> [w431 w444]
          frame False {
            n388 = Two Button Dialog(message="是否删除开机启动？" ("消息"), 1:"否" ("F按钮名称（“取消”）"), 2:"是" ("T按钮名称（“确定”）")) -> (T button?=w433:bool)
            n389 = case shown="真" w433 {
              tunnel: w432 -> [w438 _]
              tunnel: w431 -> [w437 _]
              frame False {
                n390 = property class="Bool (严格)"(reference=w438, "Value"=w437) -> ()  [unwired: 1 in, 2 out]
              }
              frame True {
                n391 = call <vilib>:"Application Directory.vi"() -> ("Application Directory"=w440:path)
                n392 = call "删除启动项.vi"("启动文件路径"=w440) -> ("删除标记"=w439:bool)  [unwired: 9 in, 1 out]
                n393 = case shown="真" w439 {
                  tunnel: ["删除开机启动失败" ("T按钮名称（“确定”）") "删除开机启动成功" ("T按钮名称（“确定”）")] -> w441
                  frame False {
                  }
                  frame True {
                  }
                }
                n394 = One Button Dialog(message=w441) -> ()  [unwired: 1 in, 1 out]
              }
            }
          }
          frame True {
            n395 = Two Button Dialog(message="是否添加开机启动？" ("消息"), 1:"否" ("F按钮名称（“取消”）"), 2:"是" ("T按钮名称（“确定”）")) -> (T button?=w446:bool)
            n396 = case shown="真" w446 {
              tunnel: w445 -> [w451 _]
              tunnel: w444 -> [w450 _]
              frame False {
                n397 = property class="Bool (严格)"(reference=w451, "Value"=w450) -> ()  [unwired: 1 in, 2 out]
              }
              frame True {
                n398 = call <vilib>:"Application Directory.vi"() -> ("Application Directory"=w454:path)
                n399 = call "添加启动项.vi"("启动文件路径"=w454) -> ("添加成功标记"=w453:bool)  [unwired: 9 in, 1 out]
                n400 = case shown="真" w453 {
                  tunnel: ["添加开机启动失败" ("T按钮名称（“确定”）") "添加开机启动成功" ("T按钮名称（“确定”）")] -> w452
                  frame False {
                  }
                  frame True {
                  }
                }
                n401 = One Button Dialog(message=w452) -> ()  [unwired: 1 in, 1 out]
              }
            }
          }
        }
      }
      event "共享MN": Value Change {
        n402 = event-data() -> ("CtlRef"=w458:refnum<vi>, "OldVal"=w457:bool, "NewVal"=w459:bool)  [unwired: 1 in, 3 out]
        n403 = case shown="真" w459 {
          tunnel: w458 -> [w461 w476]
          tunnel: w457 -> [w460 w475]
          frame False {
            n404 = Two Button Dialog(message="是否取消该MN号共享？" ("消息"), 1:"否" ("F按钮名称（“取消”）"), 2:"是" ("T按钮名称（“确定”）")) -> (T button?=w462:bool)
            n405 = case shown="真" w462 {
              tunnel: w461 -> [w467 _]
              tunnel: w460 -> [w466 _]
              frame False {
                n406 = property class="Bool (严格)"(reference=w467, "Value"=w466) -> ()  [unwired: 1 in, 2 out]
              }
              frame True {
                n407 = local read "MN"() -> (w471:string)
                n408 = local read "PW"() -> (w470:string)
                n409 = Bundle("MN"=w471, "PW"=w470) -> (w469:cluster{"MN":string, "PW":string})  [unwired: 1 in]
                n410 = call "删除MN号.vi"("簇"=w469) -> ("删除标记"=w468:bool)  [unwired: 9 in, 1 out]
                n411 = case shown="真" w468 {
                  tunnel: ["取消该MN号共享失败" ("T按钮名称（“确定”）") "取消该MN号共享成功" ("T按钮名称（“确定”）")] -> w472
                  frame False {
                  }
                  frame True {
                  }
                }
                n412 = One Button Dialog(message=w472) -> ()  [unwired: 1 in, 1 out]
              }
            }
          }
          frame True {
            n413 = Two Button Dialog(message="是否添加该MN号共享？" ("消息"), 1:"否" ("F按钮名称（“取消”）"), 2:"是" ("T按钮名称（“确定”）")) -> (T button?=w477:bool)
            n414 = case shown="真" w477 {
              tunnel: w476 -> [w482 _]
              tunnel: w475 -> [w481 _]
              frame False {
                n415 = property class="Bool (严格)"(reference=w482, "Value"=w481) -> ()  [unwired: 1 in, 2 out]
              }
              frame True {
                n416 = local read "MN"() -> (w486:string)
                n417 = local read "PW"() -> (w485:string)
                n418 = Bundle("MN"=w486, "PW"=w485) -> (w484:cluster{"MN":string, "PW":string})  [unwired: 1 in]
                n419 = call "添加MN号.vi"("簇"=w484) -> ("添加成功标记"=w483:bool)  [unwired: 9 in, 1 out]
                n420 = case shown="假" w483 {
                  tunnel: ["添加该MN号共享失败" ("T按钮名称（“确定”）") "添加该MN号共享成功" ("T按钮名称（“确定”）")] -> w487
                  frame False {
                  }
                  frame True {
                  }
                }
                n421 = One Button Dialog(message=w487) -> ()  [unwired: 1 in, 1 out]
              }
            }
          }
        }
      }
      event "更新": Value Change {
        n422 = event-data() -> ()  [unwired: 1 in, 6 out]
        n423 = call "自定义双按钮对话框.vi"("消息"="选择是否从服务器获取最新版本信息？") -> ("正式版/测试版输出"=w490:bool, "输出"=w491:bool)  [unwired: 9 in]
        n424 = case shown="真" w491 {
          tunnel: w490 -> [_ w495]
          frame False {
          }
          frame True {
            w502 = T21 2 items=["两端", "字符串首端", "字符串末端"] ("location (both)")
            w500 = "/" ("分隔符(Tab)")
            # "获取最新版本"
            n425 = local read "updateconfiguration"() -> (w506:T1)
            n426 = Unbundle By Name(w506) -> ("远程路径"=w494:string)
            n427 = Spreadsheet String To Array(delimiter (Tab)="\\" ("分隔符(Tab)"), format string="" ("格式字符串"), spreadsheet string=w494, array type (2D Dbl)=string[] []) -> (array=w497:string[])
            n428 = case shown="真" w495 {
              tunnel: w497 -> [w507 w509]
              tunnel: [w507 w508] -> w496
              frame False {
                # "正式版"
              }
              frame True {
                # "测试版"
                n429 = Array Size(array=w509) -> (size(s)=w510:i32)
                n430 = Subtract(x=w510, y=2) -> (x-y=w512:i32)
                n431 = Index Array(array=w509, index=w512) -> (element=w513:string)
                n432 = Concatenate Strings(w513, "beta" ("字符串")) -> (w515:string)
                n433 = Replace Array Subset(array=w509, new element=w515, index=w512) -> (w508:string[])
              }
            }
            n434 = Array To Spreadsheet String(delimiter (Tab)=w500, array=w496, 3:"%s" ("格式字符串")) -> (spreadsheet string=w499:string)
            n435 = Concatenate Strings(w500, w499) -> (w498:string)
            n436 = call <vilib>:"Trim Whitespace.vi"("string"=w498, "location (both)"=w502) -> ("trimmed string"=w493:string)
            n437 = call "Updateinter.vi"("更新包远端地址"=w493, "测试版？"=w495) -> ()  [unwired: 10 in]
          }
        }
      }
      event "IP", "PORT": Mouse Down {
        n438 = event-data() -> ("CtlRef"=w524:refnum<vi>)  [unwired: 1 in, 7 out]
        n439 = property class="Str"(reference=w524) -> (reference out=w522:refnum<vi>, "Value"=w523:string)  [unwired: 1 in, 1 out]
        n440 = call "IP键盘.vi"("OldNumber"=w523) -> ("NewNumber"=w519:string)
        n441 = String Length(string=w519) -> (length=w521:i32)
        n442 = Less Or Equal?(x=w521, y=50) -> (x <= y?=w518:bool)
        n443 = case shown="假" w518 {
          tunnel: w522 -> [w525 w529]
          tunnel: w519 -> [_ w528]
          tunnel: [w525 w529] -> w517
          tunnel: ["127.0.0.1" w528] -> w516
          frame False {
            n444 = One Button Dialog(message="超过ipv4最大长度限制,请重新输入!" ("消息")) -> ()  [unwired: 1 in, 1 out]
          }
          frame True {
          }
        }
        n445 = property class="Str"(reference=w517, "Val(Sgnl)"=w516) -> ()  [unwired: 1 in, 2 out]
      }
    }
  }
  n446 = while {
    shift-right: [w534] -> _
    shift-left: "数  据  采  集  传  输  系  统" ("标题显示") -> [w535]
    stop <- FALSE stop-if-true
    n447 = global read "断电保存全局.vi" "数据重发"() -> (w532:bool)
    n448 = global read "断电保存全局.vi" "日志信息重发"() -> (w531:bool)
    n449 = global read "断电保存全局.vi" "剖面数据重发"() -> (w530:bool)
    n450 = call "字符串移位显示.vi"("字符框大小"=72, "字符串输入"=w535) -> ("移位后字符串"=w534:string)  [unwired: 8 in, 1 out]
    "标题显示" <- w534
    n451 = Wait (ms)(milliseconds to wait=u32 1000 ("等待时间（毫秒）")) -> ()  [unwired: 1 out]
    n452 = property on="数据补发" class="Bool (严格)"("Visible"=w532, "Value"=w532) -> ()  [unwired: 2 in, 2 out]
    n453 = property on="日志信息补发" class="Bool (严格)"("Visible"=w531, "Value"=w531) -> ()  [unwired: 2 in, 2 out]
    n454 = property on="剖面数据补发" class="Bool (严格)"("Visible"=w530, "Value"=w530) -> ()  [unwired: 2 in, 2 out]
  }
